vi "testglobal.vi"() -> ()   [LabVIEW 2012]
panel:
  out "Boolean 2":bool
  in  "Boolean":bool
  in  "Numeric 2":dbl
  in  "Numeric":dbl
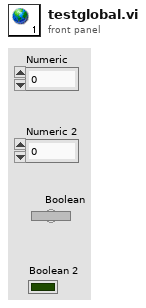
[diagram p1: front panel]
diagram:
